vi "NonlinearCharacterisation.vi"(1 "Cutoff Frequency":dbl=0.45000000000000007 format="%0.2f", 2 "Sampling Rate":dbl=1.0 format="%0.2f", 3 "Block Size":dbl=100.0, 4 "X":dbl[](graph)) -> (0 "yi":dbl[](graph))   [LabVIEW 2012]
doc: "Characterises and compensates for the static nonlinearity of a system using the assumption that the noise at its input remains constant."
uses:
  <vilib>/Analysis/3filter.llb/Filter Passband Type.ctl
  <vilib>/Analysis/6fits.llb/Curve Fitting Criteria.ctl
  <vilib>/Analysis/3filter.llb/Butterworth Filter (DBL).vi
  <vilib>/Analysis/NI_AALBase.lvlib
  <vilib>/gmath/NI_Gmath.lvlib
  <vilib>/Analysis/NI_AALPro.lvlib
panel:
  out "Transfer Function":cluster{"Y":dbl[], "Y":dbl[]}[](graph)
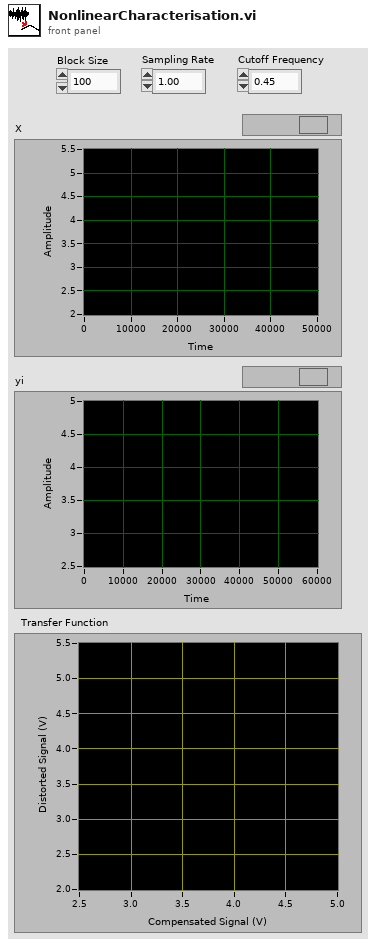
[diagram p1: front panel]
types:
  T1 = typedef "NI_AALPro.lvlib/Curve Fitting Criteria.ctl" = u16
  T2 = typedef "NI_AALBase.lvlib/Filter Passband Type.ctl" = enum32{"Lowpass", "Highpass", "Bandpass", "Bandstop"}
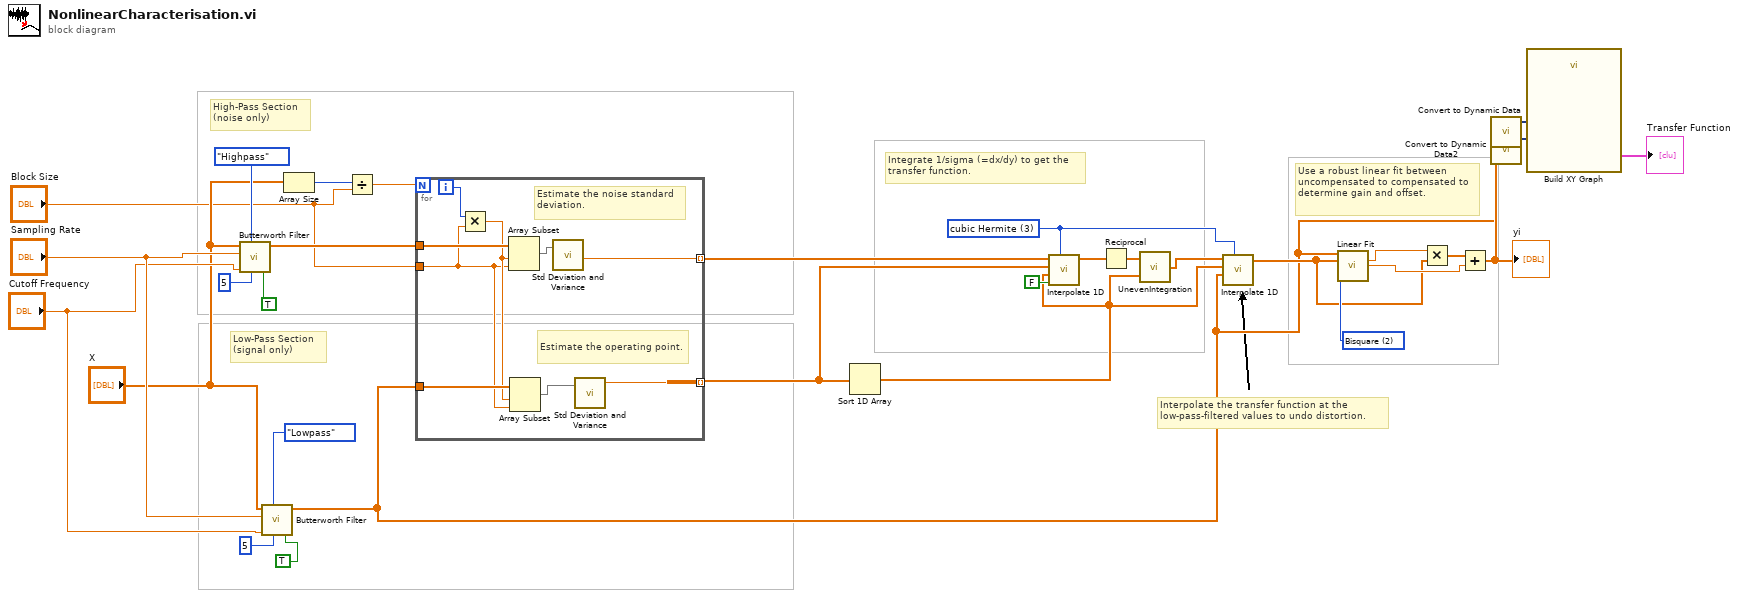
[diagram p0: block diagram]
diagram:
  w13 = 3 items=["nearest", "linear", "spline", "cubic Hermite", "Lagrange"] ("method")
  w19 = T1 2 items=["Least Square", "Least Absolute Residual", "Bisquare"] ("method")
  # "High-Pass Section\n(noise only)"
  # "Low-Pass Section\n(signal only)"
  # "Use a robust linear fit between uncompensated to compensated to determine gain and offset."
  # "Interpolate the transfer function at the\nlow-pass-filtered values to undo distortion."
  # "Integrate 1/sigma (=dx/dy) to get the\ntransfer function."
  n1 = call-poly <vilib>:"Butterworth Filter.vi"("init/cont (init:F)"=TRUE, "order"=5, "filter type"=Filter_Passband_Type."Highpass", "low cutoff freq: fl"="Cutoff Frequency", "sampling freq: fs"="Sampling Rate", "X"="X") -> ("Filtered X"=w27:dbl[])  [unwired: 2 in, 1 out]
  n2 = call-poly <vilib>:"Butterworth Filter.vi"("init/cont (init:F)"=TRUE, "order"=5, "filter type"=Filter_Passband_Type."Lowpass", "low cutoff freq: fl"="Cutoff Frequency", "sampling freq: fs"="Sampling Rate", "X"="X") -> ("Filtered X"=w2:dbl[])  [unwired: 2 in, 1 out]
  n3 = Array Size(array="X") -> (size(s)=w16:i32)
  n4 = Divide(x=w16, y="Block Size") -> (x/y=w28:dbl)
  n5 = for {
    N: w28 -> [_]
    tunnel: w27 -> [w40]
    tunnel: "Block Size" -> [w34]
    tunnel: [w32] -> w11 mode=indexing
    tunnel: w2 -> [w37]
    tunnel: [w33] -> w12 mode=indexing
    i -> [w39]
    # "Estimate the operating point."
    # "Estimate the noise standard deviation."
    n6 = Multiply(x=w39, y=w34) -> (x*y=w35:dbl)
    n7 = Array Subset(array=w40, index=w35, length=w34) -> (w38:dbl[])
    n8 = Array Subset(array=w37, index=w35, length=w34) -> (w36:dbl[])
    n9 = call <vilib>:"Std Deviation and Variance.vi"("X"=w38) -> ("standard deviation"=w32:dbl)  [unwired: 1 in, 2 out]
    n10 = call <vilib>:"Std Deviation and Variance.vi"("X"=w36) -> ("mean"=w33:dbl)  [unwired: 1 in, 2 out]
  }
  n11 = Sort 1D Array(array=w12) -> (sorted array=w5:dbl[])
  n12 = call <vilib>:"Interpolate 1D.vi"("method"=w13, "X is monotonic"=FALSE, "xi"=w5, "X"=w12, "Y"=w11) -> ("yi"=w10:dbl[])  [unwired: 4 in, 2 out]
  n13 = Reciprocal(x=w10) -> (1/x=w9:dbl[])
  n14 = call "UnevenIntegration.vi"("t"=w5, "X"=w9) -> ("Y"=w6:dbl[])
  n15 = call <vilib>:"Interpolate 1D.vi"("method"=w13, "xi"=w2, "X"=w5, "Y"=w6) -> ("yi"=w14:dbl[])  [unwired: 5 in, 2 out]
  n16 = call <vilib>:"Linear Fit.vi"("Y"=w2, "X"=w14, "method"=w19) -> ("slope"=w21:dbl, "intercept"=w20:dbl)  [unwired: 8 in, 3 out]
  n17 = Multiply(x=w21, y=w14) -> (x*y=w22:dbl[])
  n18 = Add(x=w22, y=w20) -> (x+y=w4:dbl[])
  "yi" <- w4
  n19 = call "Convert to Dynamic Data"("Array"=w4) -> ("Dynamic Data Type"=w3:dynamicdata)  [unwired: 3 in]
  n20 = call "Convert to Dynamic Data2"("Array"=w2) -> ("Dynamic Data Type"=w1:dynamicdata)  [unwired: 3 in]
  n21 = call "Build XY Graph"("Y Input"=w1, "X Input"=w3) -> ("XY Graph"=→"Transfer Function":cluster{"Y":dbl[], "Y":dbl[]}[])  [unwired: 3 in, 6 out]
